vi "Setze Zustand.vi"(6 "Zeit":sgl, 7 "Befehl nicht vorhanden!":bool, 8 "AK Befehl":string, 10 "Zustand":T1) -> (1 "Antwort String":string, 3 "Busy":bool)   [LabVIEW 2020, in "AK-Schnittstelle.lvlib"]
uses:
  AK-Schnittstelle.lvlib
  Funktionstasten/Zustaende.ctl
  Funktionstasten/Funktionstasten-Aktion.ctl
  Funktionstasten/Betriebsart.ctl
  Aktionen Zustandsfehlerinformation.ctl
  Funktionstasten/Funktionstasten.lvlib
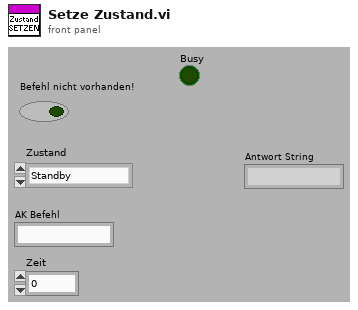
[diagram p1: front panel]
types:
  T1 = typedef "Funktionstasten.lvlib/Zustaende.ctl" = enum16{"Standby", "Pause", "Eco", "Messen", "Kalibrieren", "Spülen Filter", "Spülen Leitung", "Umgebungsluft", "0-Gas", "Cal-Gas", "CG zu PNS", "-------------", "Init 1", "Init 2", "Init 3", "Init 4", "Messen vorbereiten", "Messen durchführen", "Exit"}
  T2 = typedef "Funktionstasten.lvlib/Betriebsart.ctl" = enum16{"Manuell", "Remote", "Bitparallel"}
  T3 = typedef "Funktionstasten.lvlib/Funktionstasten-Aktion.ctl" = enum16{"Initialisieren", "Zustand setzen", "Taste gedrückt", "Fehler speichern", "Lesen", "Manuell", "Remote", "Bitparallel", "Samplepoint", "Zeit Prüfen", "reset Umschalten"}
  T4 = typedef "AK-Schnittstelle.lvlib/Aktionen Zustandsfehlerinformation.ctl" = enum16{"OK", "Offline", "Busy", "Syntax Error", "Datenfehler"}
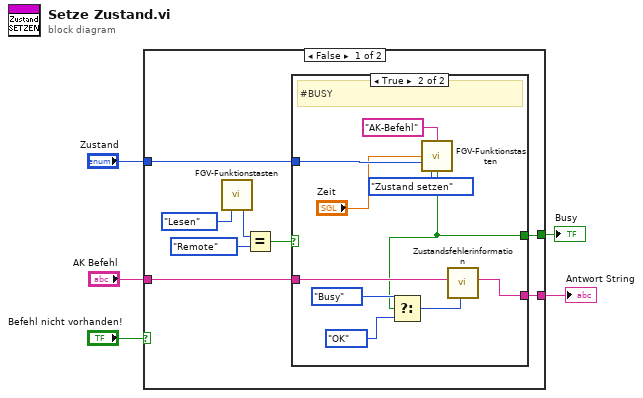
[diagram p0: block diagram]
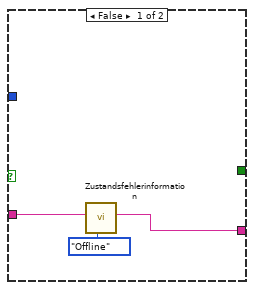
[diagram p2: hidden frame]
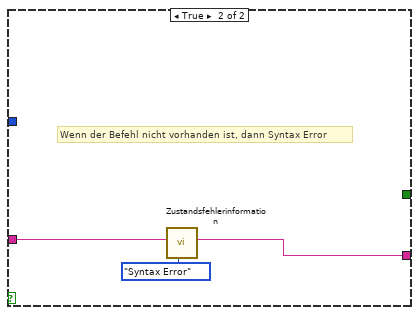
[diagram p3: hidden frame]
diagram:
  n1 = case shown="False" "Befehl nicht vorhanden!" {
    tunnel: "Zustand" -> [w13 _]
    tunnel: [w12 w27] -> w4
    tunnel: "AK Befehl" -> [w11 w28]
    tunnel: [w6 _] -> w1
    frame False {
      n2 = call "FGV-Funktionstasten.vi"("Aktion"=Funktionstasten-Aktion."Lesen") -> ("Betriebsart"=w9:T2)  [unwired: 7 in, 7 out]
      n3 = Equal?(x=w9, y=Betriebsart."Remote" ("Betriebsart")) -> (x = y?=w10:bool)
      n4 = case shown="True" w10 {
        tunnel: w11 -> [w15 w24]
        tunnel: [w14 w23] -> w12
        tunnel: w13 -> [_ w25]
        tunnel: [_ w17] -> w6
        frame False {
          n5 = call "Zustandsfehlerinformation.vi"("Aktionen"=Aktionen_Zustandsfehlerinformation."Offline", "String"=w15) -> ("String"=w14:string)  [unwired: 9 in]
        }
        frame True {
          # "#BUSY"
          n6 = call "FGV-Funktionstasten.vi"("Herkunft"="AK-Befehl", "Zeit"="Zeit", "Zustand"=w25, "Aktion"=Funktionstasten-Aktion."Zustand setzen") -> ("Busy"=w17:bool)  [unwired: 4 in, 7 out]
          n7 = Select(t=Aktionen_Zustandsfehlerinformation."Busy" ("Aktionen"), s=w17, f=Aktionen_Zustandsfehlerinformation."OK" ("Aktionen")) -> (s? t:f=w18:T4)
          n8 = call "Zustandsfehlerinformation.vi"("Aktionen"=w18, "String"=w24) -> ("String"=w23:string)  [unwired: 9 in]
        }
      }
    }
    frame True {
      # "Wenn der Befehl nicht vorhanden ist, dann Syntax Error"
      n9 = call "Zustandsfehlerinformation.vi"("Aktionen"=Aktionen_Zustandsfehlerinformation."Syntax Error", "String"=w28) -> ("String"=w27:string)  [unwired: 9 in]
    }
  }
  "Antwort String" <- w4
  "Busy" <- w1
